vi "dump_log.vi"(8 "error in (no error)":errorcluster) -> (0 "error out":errorcluster, 2 "log out":string)   [LabVIEW 2024, in "Vision.lvlib"]
uses:
  Vision.lvlib
  bin/Vision.dll
panel:
  in  "log in":string
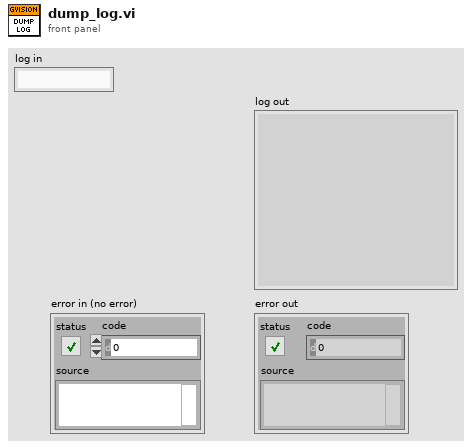
[diagram p1: front panel]
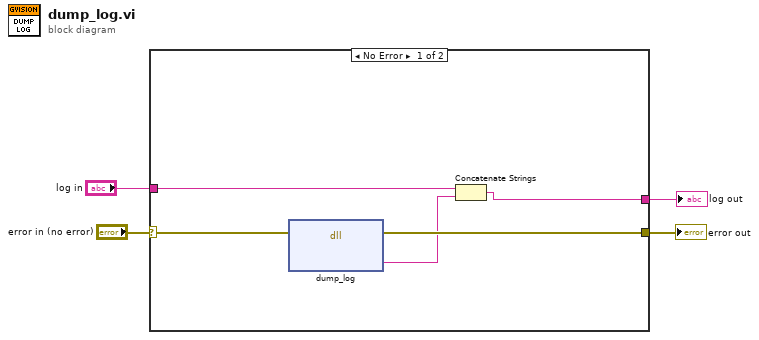
[diagram p0: block diagram]
diagram:
  n1 = case shown="No Error" "error in (no error)" {
    selector: "error in (no error)" -> [w9 w10]
    tunnel: [w8 w10] -> w3
    tunnel: [w5 _] -> w2
    tunnel: "log in" -> [w6 _]
    frame No Error {
      n2 = dll-call lib="C:/Users/cfang/Desktop/nebraska-silicon-lab/pixel-gantry-control/Gantry/Shared Components/bin/Vision.dll" fn="dump_log"(error in=w9) -> (error out=w8:errorcluster, "log"=w7:string)  [unwired: 4 in, 1 out]
      n3 = Concatenate Strings(w6, w7) -> (w5:string)
    }
    frame Error {
    }
  }
  "error out" <- w3
  "log out" <- w2
